vi "Write DAQ Queue.vi"(8 "error in (no error)":errorcluster, 10 "DAQ Queue":refnum<queue>, 11 "DAQ Interface in":refnum<class "DAQ Interface.lvclass">) -> (0 "error out":errorcluster, 3 "DAQ Interface out":refnum<class "DAQ Interface.lvclass">)   [LabVIEW 2025, in "DAQ Interface.lvlib" / "DAQ Interface.lvclass"]
uses:
  DAQ Interface.lvclass
  <vilib>/Natan Biesmans/G2CPU GPU and CPU HPC Toolkit/G2CPU Libraries/Arrays/1DArray/s16/1D Array s16.lvclass
  DAQ Interface.lvclass/DAQ Interface.ctl
  Signal Analysis/Signal Analysis/Process Data.ctl
  Signal Analysis/Signal Analysis/Signal Analysis.lvclass
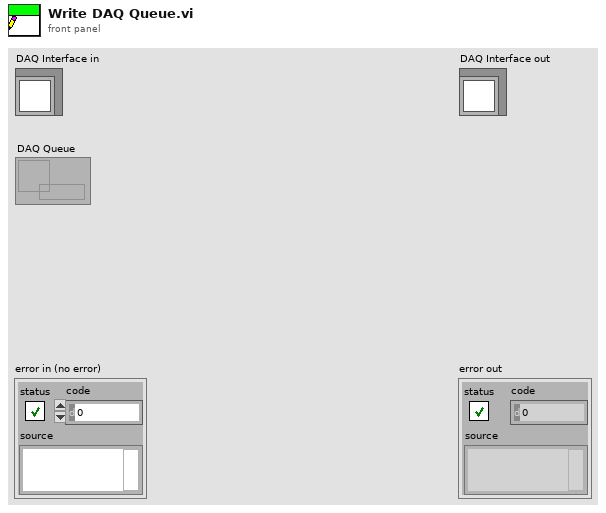
[diagram p1: front panel]
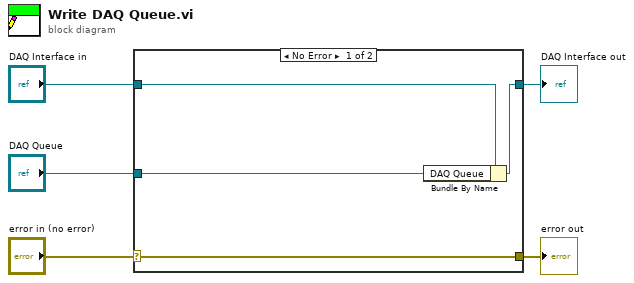
[diagram p0: block diagram]
diagram:
  n1 = case shown="No Error" "error in (no error)" {
    selector: "error in (no error)" -> [w9 w10]
    tunnel: [w9 w10] -> w4
    tunnel: [w7 w11] -> w2
    tunnel: "DAQ Interface in" -> [w8 w11]
    tunnel: "DAQ Queue" -> [w6 _]
    frame No Error {
      n2 = Bundle By Name(cluster=w8, "DAQ Queue"=w6) -> (w7:refnum<class "DAQ Interface.lvclass">)
    }
    frame Error {
    }
  }
  "error out" <- w4
  "DAQ Interface out" <- w2
